vi "Infinite Monkeys.vi"() -> ()   [LabVIEW 2015]
panel:
  in  "Show Info Popup":bool
  out "Iteration Count":u64=1965487
  in  "Text to Match":string="Rich"
  in  "stop":bool
  # "1 letter = 255"
  # "2 letter = 7k"
  # "3 letter = 1M"
  # "4 letter = 80M"
  # "5 letter = 6.1billion"
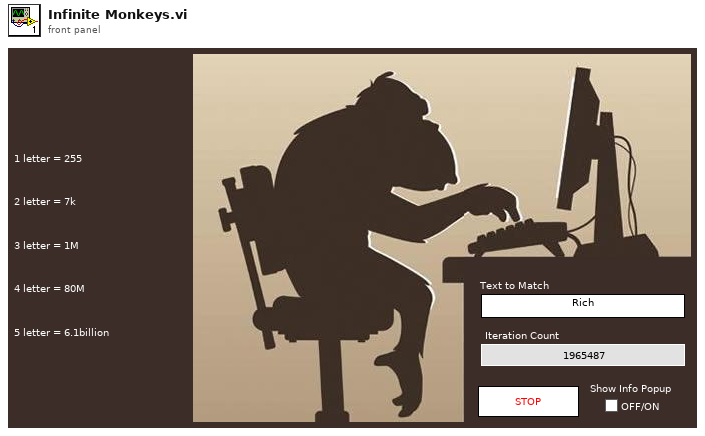
[diagram p1: front panel]
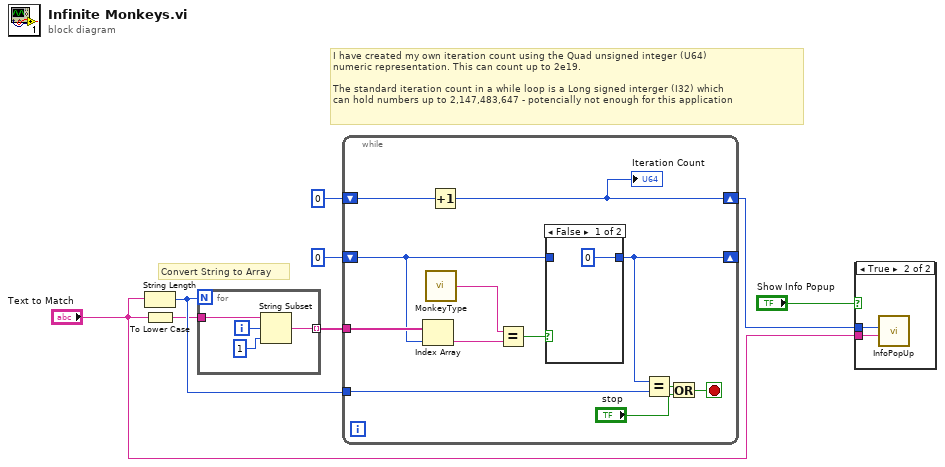
[diagram p0: block diagram]
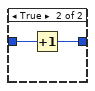
[diagram p3: hidden frame]
diagram:
  # "I have created my own iteration count using the Quad unsigned integer (U64)\nnumeric representation. This can count up to 2e19. \n\nThe standard iteration count in a while loop is a Long signed interger (I32) which\ncan hold numbers up to 2,147,483,647 - potencially not enough for this application"
  # "Convert String to Array"
  n1 = String Length(string="Text to Match") -> (length=w7:i32)
  n2 = To Lower Case(string="Text to Match") -> (all lower case string=w4:string)
  n3 = for {
    N: w7 -> [_]
    tunnel: w4 -> [w12]
    tunnel: [w9] -> w8 mode=indexing
    i -> [w10]
    n4 = String Subset(string=w12, offset (0)=w10, length (rest)=1 ("length (rest)")) -> (substring=w9:string)
  }
  n5 = while {
    tunnel: w8 -> [w24]
    shift-right: [w20] -> _
    shift-left: 0 -> [w22]
    tunnel: w7 -> [w19]
    shift-right: [w13] -> w3
    shift-left: u64 0 -> [w15]
    stop <- w18 stop-if-true
    n6 = Index Array(array=w24, index=w22) -> (element=w23:string)
    n7 = call "MonkeyType.vi"() -> ("Random Character"=w14:string)
    n8 = Increment(x=w15) -> (x+1=w13:u64)
    "Iteration Count" <- w13
    n9 = Equal?(x=w14, y=w23) -> (x = y?=w21:bool)
    n10 = case shown="False" w21 {
      tunnel: w22 -> [_ w27]
      tunnel: [0 w26] -> w20
      frame False {
      }
      frame True {
        n11 = Increment(x=w27) -> (x+1=w26:i32)
      }
    }
    n12 = Equal?(x=w20, y=w19) -> (x = y?=w17:bool)
    n13 = Or(x=w17, y="stop") -> (x .or. y?=w18:bool)
  }
  n14 = case shown="True" "Show Info Popup" {
    tunnel: w3 -> [_ w29]
    tunnel: "Text to Match" -> [_ w28]
    frame False {
    }
    frame True {
      n15 = call "InfoPopUp.vi"("Text to Match"=w28, "Iteration Count"=w29) -> ()  [unwired: 10 in]
    }
  }
